vi "Initialize Identity Attribute.vi"(11 "Name":string) -> (3 "Attribute.Identity":refnum<class "Attribute.Identity.lvclass">)   [LabVIEW 2019, in "Attribute.Identity.lvclass"]
doc: "JKI State Machine Objects (SMO) 1.3.0.56\nJKI - JKI\nCopyright (c) 2017, JKI"
uses:
  Attribute.Identity.lvclass
  Attribute.Identity.lvclass/Attribute.Identity.ctl
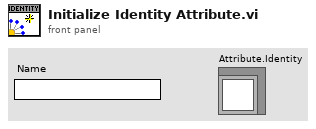
[diagram p1: front panel]
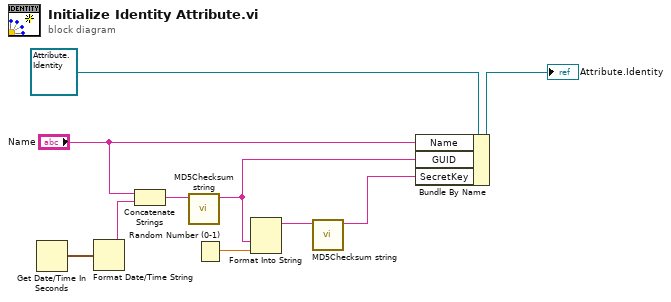
[diagram p0: block diagram]
diagram:
  n1 = Get Date/Time In Seconds() -> (seconds since 1Jan1904=w9:timestamp)
  n2 = Format Date/Time String(seconds (now)=w9) -> (date/time string=w7:string)  [unwired: 2 in]
  n3 = Concatenate Strings("Name", w7) -> (w6:string)
  n4 = call <vilib>:"MD5Checksum string.vi"("Message String"=w6) -> ("MD5 message-digest"=w4:string)  [unwired: 10 in]
  n5 = Random Number (0-1)() -> (number: 0 to 1=w5:dbl)
  n6 = Format Into String(w4, w5) -> (resulting string=w3:string)  [unwired: 3 in, 1 out]
  n7 = call <vilib>:"MD5Checksum string.vi"("Message String"=w3) -> ("MD5 message-digest"=w2:string)  [unwired: 10 in]
  n8 = Bundle By Name(cluster=refnum<class "Attribute.Identity.lvclass"> refnum ("Attribute.Owner in"), "Name"="Name", "GUID"=w4, "SecretKey"=w2) -> (→"Attribute.Identity":refnum<class "Attribute.Identity.lvclass">)
